vi "Read Status 1D.vi"(8 "error in (no error)":errorcluster, 10 "statuses in":T1[](array[typedef]) {"duration" format="%d us"}, 11 "status pointer in":refnum<class "Status.lvclass">) -> (0 "error out":errorcluster, 2 "statuses out":T1[](array[typedef]) {"duration" format="%d us"}, 3 "status pointer out":refnum<class "Status.lvclass">)   [LabVIEW 2017, in "DSF Core.lvlib" / "Status.lvclass"]
uses:
  Status.lvclass
  C:/Program Files (x86)/National Instruments/LabVIEW 2017/vi.lib/NI/Memory Manager/Classes/Pointer/Pointer.lvclass
  Status Data.ctl
  <vilib>/NI/Memory Manager/Classes/Pointer/Pointer.lvclass/Pointer.ctl
  <vilib>/NI/Memory Manager/Classes/Pointer/Errors.vi
  <vilib>/NI/Memory Manager/Classes/Pointer/Null Pointer.vi
  <vilib>/NI/Memory Manager/Classes/Pointer/Is Null.vi
  <vilib>/NI/Memory Manager/Classes/Pointer/Out of Bounds.vi
  <vilib>/NI/Memory Manager/Classes/Pointer/Get Size.vi
  <vilib>/NI/Memory Manager/Classes/Pointer/Create Error.vi
  <vilib>/NI/Memory Manager/Classes/Pointer/Write Pointer Size to Error.vi
  <vilib>/NI/Memory Manager/Constants/Constants.vi
  <vilib>/NI/Memory Manager/Constants/Library Name.vi
  <vilib>/NI/Memory Manager/Classes/Pointer/Pointer Error Info.vi
  <vilib>/NI/Memory Manager/Constants/Pointer Class Name.vi
  <vilib>/NI/Memory Manager/VIs/New Error Cluster.vi
  <vilib>/NI/Memory Manager/VIs/New Error Cluster (512B).vi
  <vilib>/NI/Memory Manager/VIs/Set Error Status.vi
  <vilib>/NI/Memory Manager/VIs/Set Error Code.vi
  <vilib>/NI/Memory Manager/VIs/Set Error Source.vi
  <vilib>/NI/Memory Manager/VIs/Write String to Source.vi
  <vilib>/NI/Memory Manager/VIs/Write Numeric to Source.vi
  <vilib>/NI/Memory Manager/VIs/Write Numeric Scalar to Source (Base10 U64).vi
  <vilib>/NI/Memory Manager/Classes/Pointer/Pointer.lvclass
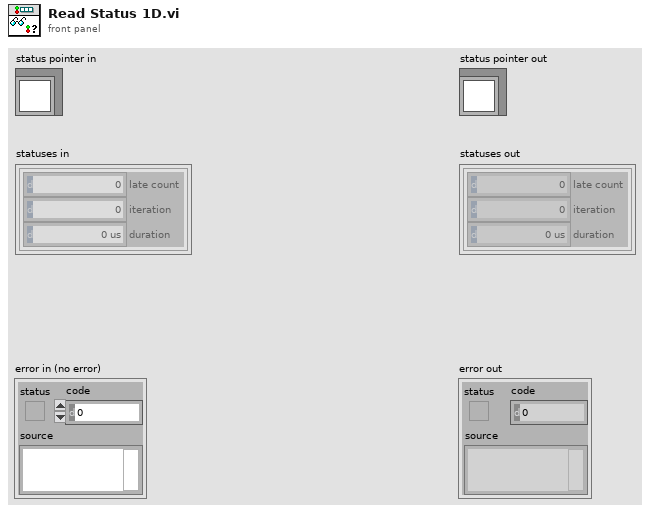
[diagram p1: front panel]
types:
  T1 = typedef "DSF Core.lvlib/Status.lvclass/Status Data.ctl" = cluster{"late count":u64, "iteration":u64, "duration":u32}
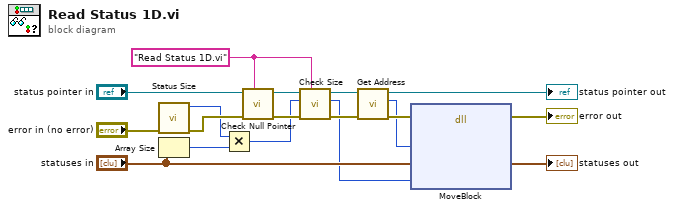
[diagram p0: block diagram]
diagram:
  w1 = "Read Status 1D.vi" ("source vi name")
  n1 = call "Status Size.vi"("error in (no error)"="error in (no error)") -> ("error out"=w12:errorcluster, "size"=w11:u64)  [unwired: 9 in]
  n2 = Array Size(array="statuses in") -> (size(s)=w10:i32)
  n3 = Multiply(x=w11, y=w10) -> (x*y=w2:u64)
  n4 = call <vilib>:"Check Null Pointer.vi"("source vi name"=w1, "error in (no error)"=w12, "Pointer in"="status pointer in") -> ("error out"=w13:errorcluster, "Pointer out"=w15:refnum<class "Status.lvclass">)  [unwired: 7 in]
  n5 = call <vilib>:"Check Size.vi"("source vi name"=w1, "error in (no error)"=w13, "required size"=w2, "Pointer in"=w15) -> ("error out"=w7:errorcluster, "required size out"=w4:u64, "Pointer out"=w14:refnum<class "Status.lvclass">)  [unwired: 5 in]
  n6 = call <vilib>:"Get Address.vi"("Pointer in"=w14) -> ("address"=w3:u64, "Pointer out"=→"status pointer out":refnum<class "Status.lvclass">)  [unwired: 9 in]
  n7 = dll-call lib="LabVIEW" fn="MoveBlock"(error in=w7, "src"=w3, "dst"="statuses in", "size"=w4) -> (error out=→"error out":errorcluster, "dst"=→"statuses out":T1[])  [unwired: 5 in, 1 out]
